vi "Configure AMQP Client.vi"(8 "error in (no error)":errorcluster, 11 "Logger in":refnum<class "Logger.lvclass">) -> (0 "error out":errorcluster, 3 "Logger out":refnum<class "Logger.lvclass">)   [LabVIEW 2017, in "Logger.lvlib" / "Logger.lvclass"]
uses:
  Logger.lvclass
  Logger.lvclass/Logger.ctl
  <vilib>/Skyline/Configuration/Configuration AMQP_class/Open Configuration AMQP.vi
  <vilib>/Skyline/Configuration/Configuration_class/NI Skyline Configuration.lvclass
  <vilib>/Skyline/Configuration/Configuration AMQP_class/NI Skyline Configuration AMQP.lvclass
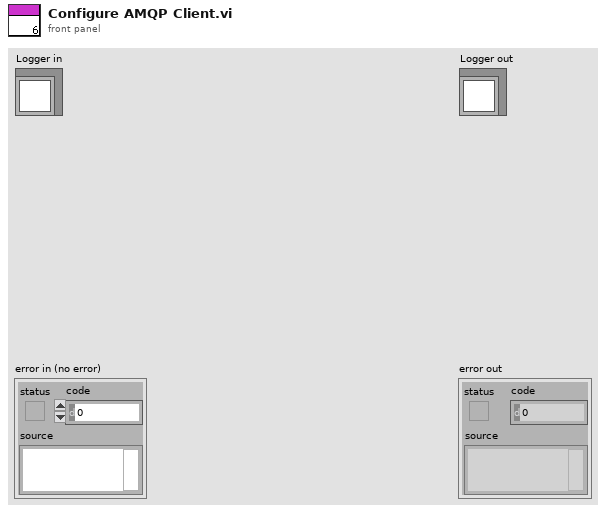
[diagram p1: front panel]
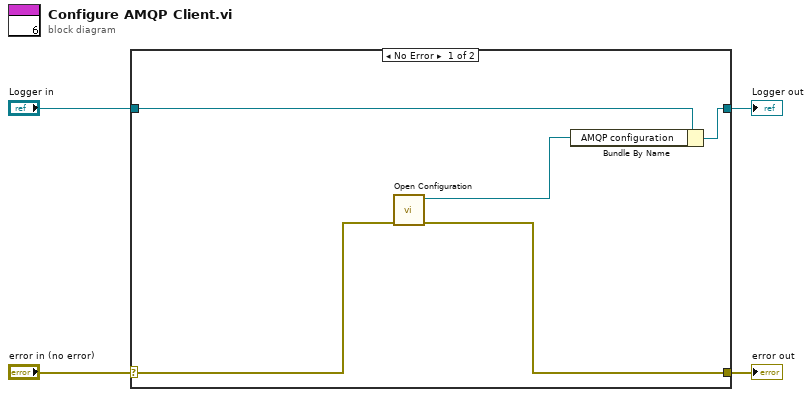
[diagram p0: block diagram]
diagram:
  n1 = case shown="No Error" "error in (no error)" {
    selector: "error in (no error)" -> [w6 w11]
    tunnel: [w5 w11] -> w3
    tunnel: [w7 w10] -> w1
    tunnel: "Logger in" -> [w9 w10]
    frame No Error {
      n2 = call-poly <vilib>:"Open Configuration.vi"("error in (no error)"=w6) -> ("error out"=w5:errorcluster, "AMQP configuration out"=w8:refnum<class "NI Skyline Configuration AMQP.lvclass">)  [unwired: 9 in]
      n3 = Bundle By Name(cluster=w9, "AMQP configuration"=w8) -> (w7:refnum<class "Logger.lvclass">)
    }
    frame Error {
    }
  }
  "error out" <- w3
  "Logger out" <- w1
